vi "Copy_API_ID.vi"(1 "Input List":cluster{string, string[], dbl[], dbl}[](array[cluster]), 2 "Input Sequence":cluster{string, string[], dbl[], dbl}[](array[cluster])) -> (0 "Output List":cluster{string, string[], dbl[], dbl}[](array[cluster]))   [LabVIEW 2011]
doc: "This VI is used when copying API events. Every API Event start/end pair has a unique ID. The \"Input List\" parameter should contain all newly created events that should be copied. This VI will assign new API ID's to these events, so as not to conflict with the existing events in the \"Input Sequence\"."
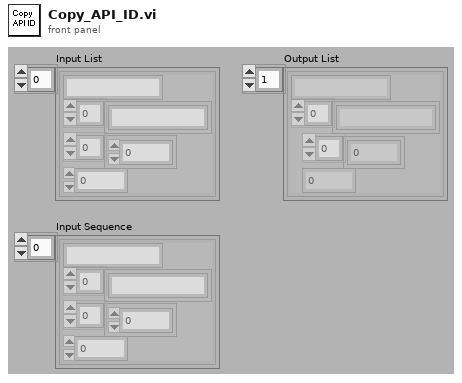
[diagram p1: front panel]
types:
  T1 = cluster{string, "Argument List Out":string[], dbl[], dbl}
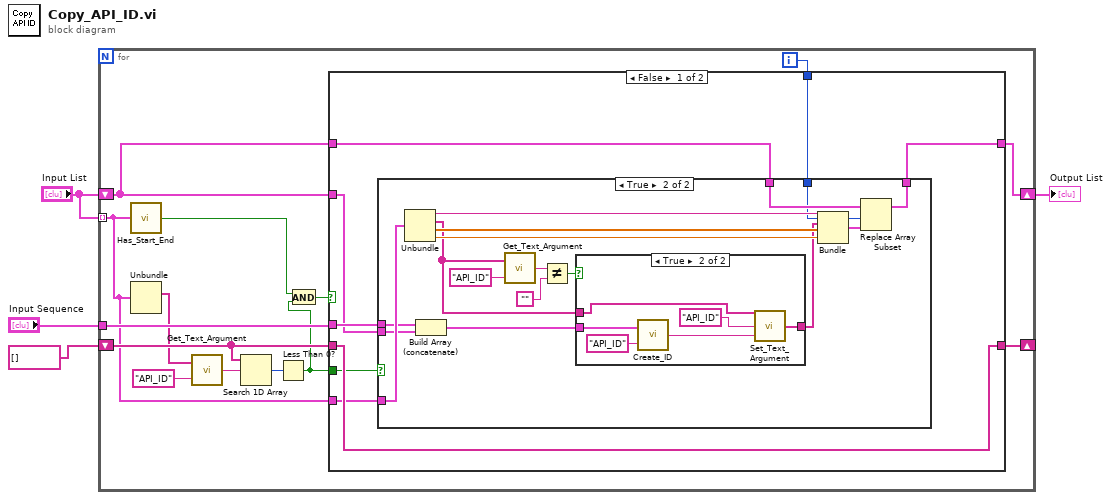
[diagram p0: block diagram]
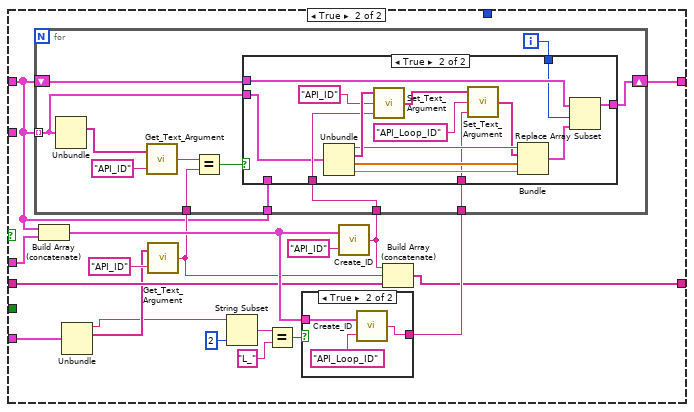
[diagram p4: hidden frame]
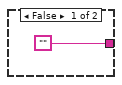
[diagram p5: hidden frame]
diagram:
  n1 = for {
    tunnel: "Input List" -> [w9] mode=indexing
    tunnel: "Input Sequence" -> [w18]
    shift-right: [w17] -> _
    shift-left: string[] [] -> [w15]
    shift-right: [w7] -> w1
    shift-left: "Input List" -> [w5]
    i -> [w6]
    n2 = call "Has_Start_End.vi"("Command"=w9) -> ("Has Start and End"=w8:bool)
    n3 = Unbundle(w9) -> (w10:string[])  [unwired: 3 out]
    n4 = call "Get_Text_Argument.vi"("Argument"="API_ID", "Argument List"=w10) -> ("Text"=w14:string)
    n5 = Search 1D Array(1D array=w15, element=w14) -> (index of element=w13:i32)  [unwired: 1 in]
    n6 = Less Than 0?(x=w13) -> (x < 0?=w11:bool)
    n7 = And(x=w8, y=w11) -> (x .and. y?=w12:bool)
    n8 = case shown="False" w12 {
      tunnel: w18 -> [w24 w54]
      tunnel: [w26 w60] -> w17
      tunnel: w15 -> [w26 w59]
      tunnel: w5 -> [w21 w52]
      tunnel: w9 -> [w25 w58]
      tunnel: w11 -> [w22 _]
      tunnel: [w19 w53] -> w7
      tunnel: w6 -> [w20 _]
      tunnel: w5 -> [w23 _]
      frame False {
        n9 = case shown="True" w22 {
          tunnel: w25 -> [_ w44]
          tunnel: w24 -> [_ w43]
          tunnel: w23 -> [_ w37]
          tunnel: w21 -> [w27 w36]
          tunnel: w20 -> [_ w35]
          tunnel: [w27 w33] -> w19
          frame False {
          }
          frame True {
            n10 = Unbundle(w44) -> (w42:string, w31:string[], w41:dbl[], w40:dbl)
            n11 = Build Array (concatenate)(w43, w37) -> (w39:cluster{string, string[], dbl[], dbl}[])
            n12 = call "Get_Text_Argument.vi"("Argument"="API_ID", "Argument List"=w31) -> ("Text"=w30:string)
            n13 = Not Equal?(x=w30, y="") -> (x != y?=w28:bool)
            n14 = case shown="True" w28 {
              tunnel: w39 -> [_ w50]
              tunnel: w31 -> [w45 w47]
              tunnel: [w45 w46] -> w38
              frame False {
              }
              frame True {
                n15 = call "Create_ID.vi"("ID Argument Name"="API_ID", "Input Sequence"=w50) -> ("ID"=w48:string)
                n16 = call "Set_Text_Argument.vi"("Text"=w48, "Argument"="API_ID", "Argument List In"=w47) -> ("Argument List Out"=w46:string[])
              }
            }
            n17 = Bundle(w42, "Argument List Out"=w38, w41, w40) -> (w34:T1)  [unwired: 1 in]
            n18 = Replace Array Subset(array=w36, new element=w34, index=w35) -> (w33:cluster{string, string[], dbl[], dbl}[])
          }
        }
      }
      frame True {
        n19 = Build Array (concatenate)(w52, w54) -> (w62:cluster{string, string[], dbl[], dbl}[])
        n20 = Unbundle(w58) -> (w56:string, w57:string[])  [unwired: 2 out]
        n21 = call "Get_Text_Argument.vi"("Argument"="API_ID", "Argument List"=w57) -> ("Text"=w61:string)
        n22 = String Subset(string=w56, length (rest)=2 ("length (rest)")) -> (substring=w67:string)  [unwired: 1 in]
        n23 = Equal?(x=w67, y="L_") -> (x = y?=w65:bool)
        n24 = case shown="True" w65 {
          tunnel: w62 -> [_ w73]
          tunnel: ["" w72] -> w64
          frame False {
          }
          frame True {
            n25 = call "Create_ID.vi"("ID Argument Name"="API_Loop_ID", "Input Sequence"=w73) -> ("ID"=w72:string)
          }
        }
        n26 = call "Create_ID.vi"("ID Argument Name"="API_ID", "Input Sequence"=w62) -> ("ID"=w55:string)
        n27 = for {
          tunnel: w52 -> [w78] mode=indexing
          tunnel: w61 -> [w85]
          tunnel: w52 -> [w84]
          tunnel: w55 -> [w83]
          tunnel: w64 -> [w81]
          shift-right: [w80] -> w53
          shift-left: w52 -> [w79]
          i -> [w74]
          n28 = Unbundle(w78) -> (w82:string[])  [unwired: 3 out]
          n29 = call "Get_Text_Argument.vi"("Argument"="API_ID", "Argument List"=w82) -> ("Text"=w76:string)
          n30 = Equal?(x=w76, y=w85) -> (x = y?=w75:bool)
          n31 = case shown="True" w75 {
            tunnel: w84 -> [_ _]
            tunnel: w83 -> [_ w96]
            tunnel: w81 -> [_ w93]
            tunnel: w79 -> [w86 w90]
            tunnel: [w86 w89] -> w80
            tunnel: w78 -> [_ w91]
            tunnel: w74 -> [_ w88]
            frame False {
            }
            frame True {
              n32 = Unbundle(w91) -> (w100:string, w101:string[], w99:dbl[], w98:dbl)
              n33 = call "Set_Text_Argument.vi"("Text"=w96, "Argument"="API_ID", "Argument List In"=w101) -> ("Argument List Out"=w95:string[])
              n34 = call "Set_Text_Argument.vi"("Text"=w93, "Argument"="API_Loop_ID", "Argument List In"=w95) -> ("Argument List Out"=w92:string[])
              n35 = Bundle(w100, "Argument List Out"=w92, w99, w98) -> (w87:T1)  [unwired: 1 out]
              n36 = Replace Array Subset(array=w90, new element=w87, index=w88) -> (w89:cluster{string, string[], dbl[], dbl}[])
            }
          }
        }
        n37 = Build Array (concatenate)(w55, w61, w59) -> (w60:string[])
      }
    }
  }
  "Output List" <- w1
